vi "Command-DestroyWindow.vi"(8 "error in (no error)":errorcluster, 10 "Data":T1, 11 "Engine in":refnum<class "Engine.lvclass">) -> (3 "Engine out":refnum<class "Engine.lvclass">)   [LabVIEW 2020, in "GLF.lvlib" / "Engine.lvclass"]
uses:
  Engine.lvclass
  Window/Window.lvclass
  Engine.lvclass/Engine.ctl
  Command-DestroyWindow--cluster.ctl
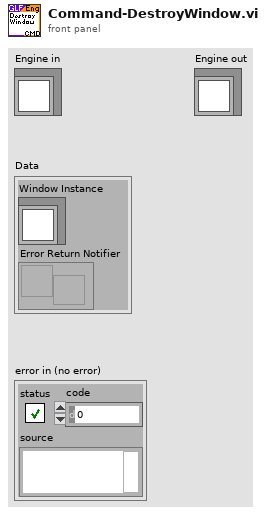
[diagram p1: front panel]
types:
  T1 = typedef "GLF.lvlib/Engine.lvclass/Command-DestroyWindow--cluster.ctl" = cluster{"Window Instance":refnum<class "Window.lvclass">, "Error Return Notifier":refnum<notifier>}
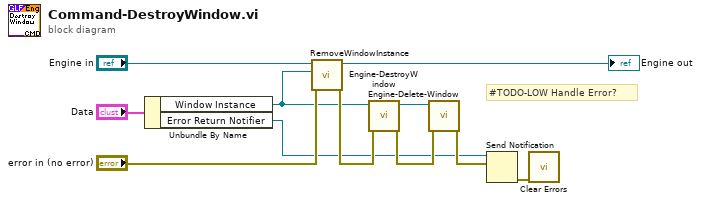
[diagram p0: block diagram]
diagram:
  # "#TODO-LOW Handle Error?"
  n1 = Unbundle By Name("Data") -> ("Window Instance"=w5:refnum<class "Window.lvclass">, "Error Return Notifier"=w1:refnum<notifier>)
  n2 = call "RemoveWindowInstance.vi"("error in (no error)"="error in (no error)", "Window Instance"=w5, "Engine in"="Engine in") -> ("error out"=w11:errorcluster, "Engine out"=→"Engine out":refnum<class "Engine.lvclass">)  [unwired: 7 in]
  n3 = call "Engine-DestroyWindow.vi"("error in (no error)"=w11, "Window in"=w5) -> ("error out"=w3:errorcluster, "Window out"=w4:refnum<class "Window.lvclass">)  [unwired: 8 in]
  n4 = call "Engine-Delete-Window.vi"("error in (no error)"=w3, "Window in"=w4) -> ("error out"=w2:errorcluster)  [unwired: 9 in]
  n5 = Send Notification(notification=w2, notifier=w1) -> (error out=w8:errorcluster)  [unwired: 1 in, 1 out]
  n6 = call <vilib>:"Clear Errors.vi"("error in (no error)"=w8) -> ()  [unwired: 5 in, 2 out]
